vi "TimePressed2DistTraveled.vi"(2 "num_timeToTravel":i64, 3 "num_velocity":i64) -> (7 "num_distTraveled":i64)   [LabVIEW 2022 SP3]
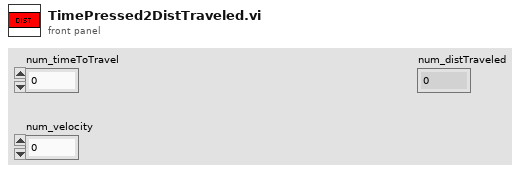
[diagram p1: front panel]
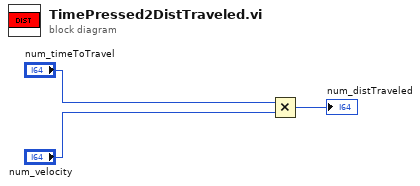
[diagram p0: block diagram]
diagram:
  n1 = Multiply(x="num_timeToTravel", y="num_velocity") -> (x*y=→"num_distTraveled":i64)
